vi "Load Animation.vi"(8 "Error In":errorcluster, 9 "Position":cluster{"X":i16, "Y":i16}, 10 "FPS":u32=30) -> (0 "Error Out":errorcluster, 3 "Animation Congig":T1)   [LabVIEW 2011, in "LVH-Toolbox.lvlib" / "LVH-SystemTools.lvlib"]
uses:
  LVH-SystemTools.lvlib
  Private/UI/Animations/Animation Config.ctl
  <vilib>/picture/picture.llb/imagedata.ctl
  Private/UI/Type Defs/FGV States.ctl
panel:
  out "call chain":string[](array[string])
  in  "Animation":enum16{"Green Bars"}(ring)
  in  "Animation Config":T1
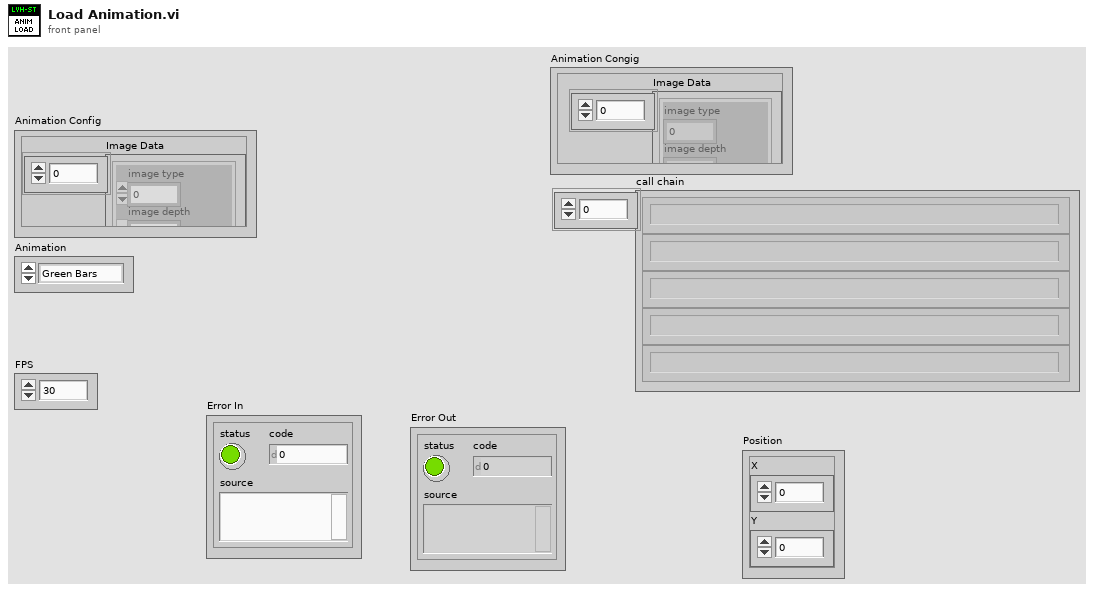
[diagram p1: front panel]
types:
  T1 = typedef "LVH-Toolbox.lvlib/LVH-SystemTools.lvlib/Animation Config.ctl" = cluster{"Image Data":T2[], "FPS":u32, "Position":cluster{"X":i16, "Y":i16}}
  T2 = typedef "imagedata.ctl" = cluster{"image type":i32, "image depth":i32, "image":u8[], "mask":u8[], "colors":u32[], "Rectangle":cluster{"left":i16, "top":i16, "right":i16, "bottom":i16}}
  T3 = typedef "LVH-Toolbox.lvlib/LVH-SystemTools.lvlib/FGV States.ctl" = enum16{"Init", "Set", "Get"}
  T4 = typedef "LVRectTypeDef.ctl" = cluster{"left":i16, "top":i16, "right":i16, "bottom":i16}
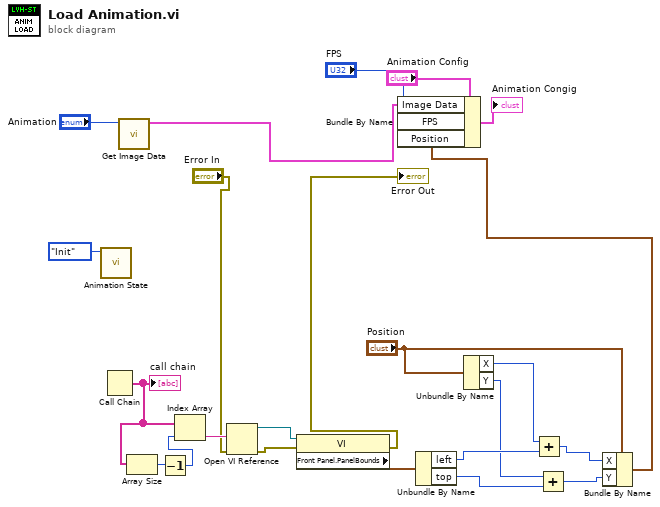
[diagram p0: block diagram]
diagram:
  n1 = call "Animation State.vi"("Function"=FGV_States."Init") -> ()  [unwired: 10 in, 1 out]
  n2 = Call Chain() -> (call chain=w15:string[])
  "call chain" <- w15
  n3 = call "Get Image Data.vi"("Animation"="Animation") -> ("Frame Data"=w18:T2[])  [unwired: 10 in]
  n4 = Array Size(array=w15) -> (size(s)=w17:i32)
  n5 = Decrement(x=w17) -> (x-1=w16:i32)
  n6 = Index Array(array=w15, index=w16) -> (element=w14:string)
  n7 = Open VI Reference(vi path=w14, error in (no error)="Error In") -> (vi reference=w13:refnum<vi>, error out=w12:errorcluster)  [unwired: 4 in]
  n8 = property class="VI"(reference=w13, error in=w12) -> (error out=→"Error Out":errorcluster, "Front Panel.PanelBounds"=w11:T4)  [unwired: 1 out]
  n9 = Unbundle By Name(w11) -> ("left"=w9:i16, "top"=w7:i16)
  n10 = Unbundle By Name("Position") -> ("X"=w10:i16, "Y"=w8:i16)
  n11 = Add(x=w10, y=w9) -> (x+y=w6:i16)
  n12 = Add(x=w8, y=w7) -> (x+y=w5:i16)
  n13 = Bundle By Name(cluster="Position", "X"=w6, "Y"=w5) -> (w3:cluster{"X":i16, "Y":i16})
  n14 = Bundle By Name(cluster="Animation Config", "Image Data"=w18, "FPS"="FPS", "Position"=w3) -> (→"Animation Congig":T1)
